vi "Measurement Logic2.vi"(8 "error in":errorcluster, 9 "measurement configuration":T2={"Capturing Stream"=FALSE, "Pause Capture In"=FALSE, "Interface Name In"="ENET9/monitor", "Update Interval s in"=0.2, "Packet Count"=0}, 10 "measure call context in":refnum<class "Measure Call Context.lvclass">) -> (0 "error out":errorcluster, 1 "measurement results":T1={"Dataframe"=[[""]], "Capturing Stream"=TRUE, "Packet Count Out"=0}, 2 "measure call context out":refnum<class "Measure Call Context.lvclass">)   [LabVIEW 2025, in "Automotive Ethernet Bus Monitor.lvclass"]
doc: "Contains the core logic for executing the measurement."
uses:
  Automotive Ethernet Bus Monitor.lvclass
  <vilib>/Plug-In SDKs/Measurements/Measure Call Context/Measure Call Context.lvclass
  Measurement Configuration.ctl
  Measurement Results.ctl
  <vilib>/xnet/xnet.llb/XNET Create Session (Frame Input Stream).vi
  <vilib>/xnet/xnet.llb/XNET Read (Frame Ethernet).vi
  <extravilib>/ChannelInstances/Event Messenger-bool/Instantiate.vi
  Automotive Ethernet Bus Monitor.lvclass/Automotive Ethernet Bus Monitor.ctl
  Program Files/NI/LVAddons/nixnet/1/examples/nixnet/projects/NI-XNET Ethernet/subVI/Ethernet.lvlib
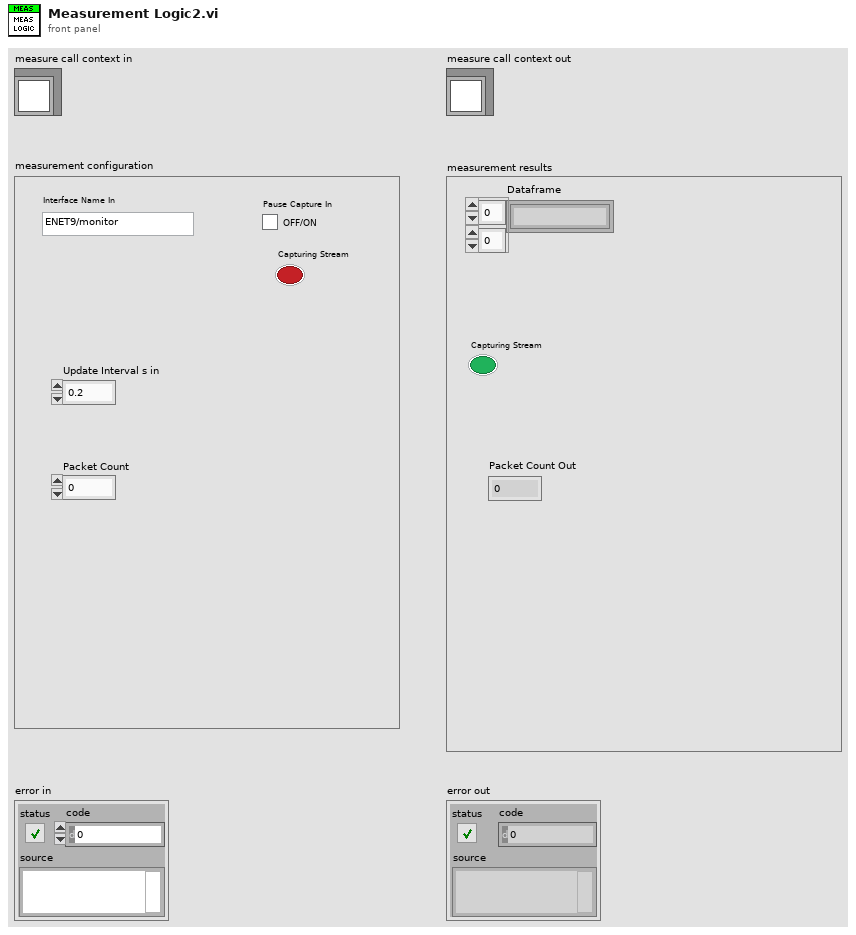
[diagram p1: front panel]
types:
  T1 = typedef "Automotive Ethernet Bus Monitor.lvclass/Measurement Results.ctl" = cluster{"Dataframe":string[][], "Capturing Stream":bool, "Packet Count Out":u32}
  T2 = typedef "Automotive Ethernet Bus Monitor.lvclass/Measurement Configuration.ctl" = cluster{"Capturing Stream":bool, "Pause Capture In":bool, "Interface Name In":string, "Update Interval s in":dbl, "Packet Count":u32}
  T3 = typedef "XNET Frame Ethernet.ctl" = cluster{"local timestamp":timestamp, "network timestamp":timestamp, "frame data":u8[], "fcs":u32, "type":T4, "network synced?":bool, "receive?":bool, "transmit?":bool, "error?":bool}
  T4 = typedef "XNET Frame Type Ethernet.ctl" = u16
  T5 = typedef "Ethernet.lvlib/Ethernet Header.ctl" = cluster{"destination MAC address":cluster{u8, u8, u8, u8, u8, u8}, "source MAC address":cluster{u8, u8, u8, u8, u8, u8}, "Has VLAN Tag":bool, "VLAN Tag":T6, "Ethertype":u16}
  T6 = typedef "Ethernet.lvlib/VLAN Tag.ctl" = cluster{"TPID":u16, "priority":u8, "DEI":bool, "VID":u16}
  T7 = typedef "Event Messenger-bool.lvlib/))Channel.ctl" = refnum<queue>
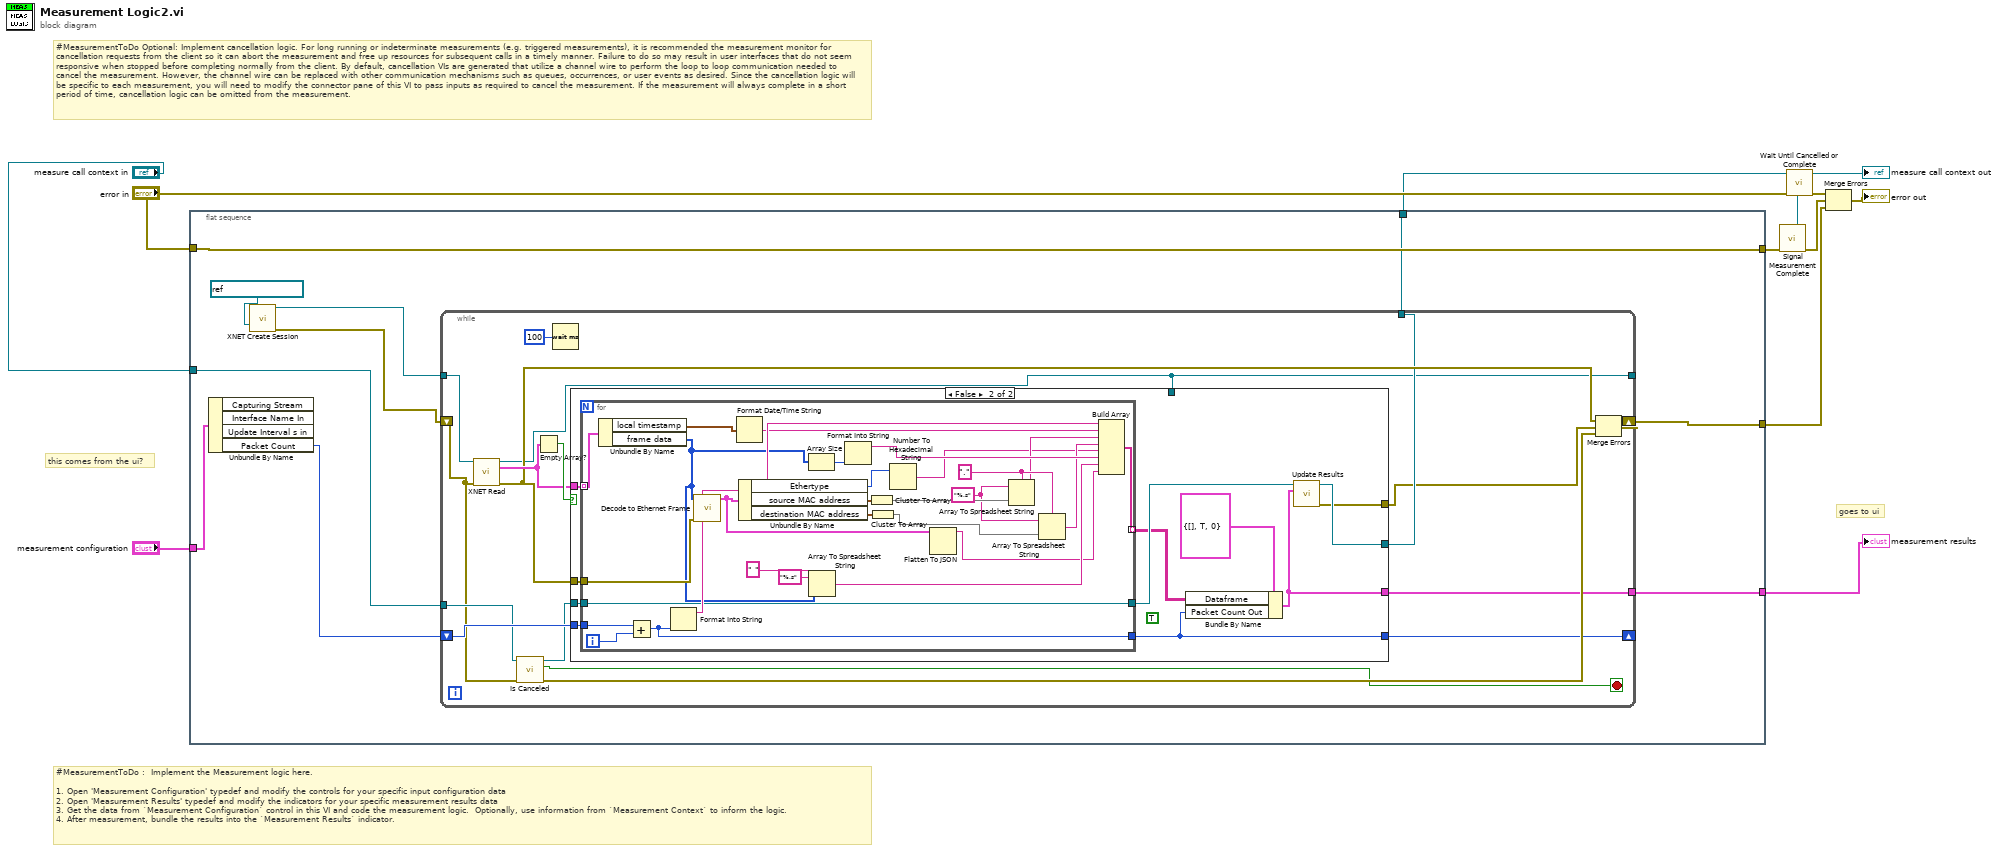
[diagram p0: block diagram]
diagram:
  # "goes to ui"
  # "this comes from the ui?"
  # "#MeasurementToDo Optional: Implement cancellation logic. For long running or indeterminate measurements (e.g. triggered measurements), it is recommended the measurement monitor for cancellation requests from the client so it can abort the measurement and free up resources for subsequent calls in a timely manner. Failure to do so may result in user interfaces that do not seem responsive when stopped before completing normally from the client. By default, cancellation VIs are generated that utilize a channel wire to perform the loop to loop communication needed to cancel the measurement. However, the channel wire can be replaced with other communication mechanisms such as queues, occurrences, or user events as desired. Since the cancellation logic will be specific to each measurement, you will need to modify the connector pane of this VI to pass inputs as required to cancel the measurement. If the measurement will always complete in a short period of time, cancellation logic can be omitted from the measurement."
  # "#MeasurementToDo :  Implement the Measurement logic here.\n\n1. Open 'Measurement Configuration' typedef and modify the controls for your specific input configuration data\n2. Open 'Measurement Results' typedef and modify the indicators for your specific measurement results data\n3. Get the data from `Measurement Configuration` control in this VI and code the measurement logic.  Optionally, use information from `Measurement Context` to inform the logic.\n4. After measurement, bundle the results into the `Measurement Results` indicator."
  n1 = flat-sequence {
    tunnel: "measurement configuration" -> [w21]
    tunnel: "error in" -> [w22]
    tunnel: [w22] -> w9
    tunnel: "measure call context in" -> [w18]
    tunnel: [w17] -> w3
    tunnel: [w16] -> w2
    tunnel: [w14] -> w1
    frame #0 {
      n2 = Unbundle By Name(w21) -> ("Packet Count"=w20:u32)  [unwired: 3 out]
      n3 = call-poly <vilib>:"XNET Create Session.vi"("interface"=refnum<k21> "ENET9/monitor") -> ("session out"=w15:refnum<k21>, "error out"=w13:errorcluster)  [unwired: 13 in]
      n4 = while {
        tunnel: w15 -> [w37]
        tunnel: [w25] -> _
        shift-right: [w26] -> _
        shift-left: w20 -> [w36]
        tunnel: w18 -> [w33]
        tunnel: [w30] -> w17
        tunnel: [w24] -> w14
        shift-right: [w34] -> w16
        shift-left: w13 -> [w23]
        stop <- w29 stop-if-true
        n5 = call-poly <vilib>:"XNET Read.vi"("session in"=w37, "error in (no error)"=w23) -> ("session out"=w25:refnum<k21>, "data"=w38:T3[], "error out"=w35:errorcluster)  [unwired: 10 in, 1 out]
        n6 = call <vilib>:"Is Canceled.vi"("error in"=w23, "measure call context in"=w33) -> ("error out"=w31:errorcluster, "is canceled?"=w29:bool, "measure call context out"=w32:refnum<class "Measure Call Context.lvclass">)  [unwired: 7 in]
        n7 = Empty Array?(array=w38) -> (empty?=w39:bool)
        n8 = Wait (ms)(milliseconds to wait=u32 100) -> ()  [unwired: 1 out]
        n9 = case shown="False" w39 {
          tunnel: w38 -> [_ w53]
          tunnel: w36 -> [w42 w52]
          tunnel: [w42 w45] -> w26
          tunnel: [w41 w49] -> w30
          tunnel: w35 -> [w40 w51]
          tunnel: w32 -> [w41 w50]
          tunnel: [w40 w48] -> w28
          tunnel: w25 -> [_ _]
          tunnel: [_ w44] -> w24
          frame True {
          }
          frame False {
            (unwired) TRUE ("Capturing Stream")
            n10 = for {
              tunnel: w53 -> [w81] mode=indexing
              tunnel: w52 -> [w72]
              tunnel: [w71] -> w45
              tunnel: w51 -> [w69]
              tunnel: w50 -> [w70]
              tunnel: [w70] -> w47
              tunnel: [w68] -> w43 mode=indexing
              i -> [w73]
              w64 = "%.s" ("format string")
              w65 = "." ("delimiter (Tab)")
              n11 = Unbundle By Name(w81) -> ("local timestamp"=w80:timestamp, "frame data"=w59:u8[])
              n12 = Add(x=w72, y=w73) -> (x+y=w71:u32)
              n13 = Format Into String(w71) -> (resulting string=w79:string)  [unwired: 3 in, 1 out]
              n14 = call "Decode to Ethernet Frame.vi"("error in (no error)"=w69, "frame data"=w59) -> ("Ethernet Header Cluster"=w54:T5)  [unwired: 7 in, 2 out]
              n15 = Format Date/Time String(seconds (now)=w80) -> (date/time string=w76:string)  [unwired: 2 in]
              n16 = Unbundle By Name(w54) -> ("Ethertype"=w56:u16, "source MAC address"=w78:cluster{u8, u8, u8, u8, u8, u8}, "destination MAC address"=w77:cluster{u8, u8, u8, u8, u8, u8})
              n17 = Array Size(array=w59) -> (size(s)=w75:i32)
              n18 = Array To Spreadsheet String(delimiter (Tab)=" ", array=w59, 3:"%.s" ("format string")) -> (spreadsheet string=w58:string)
              n19 = Format Into String(w75) -> (resulting string=w74:string)  [unwired: 3 in, 1 out]
              n20 = Cluster To Array(cluster=w78) -> (array=w67:u8[])
              n21 = Cluster To Array(cluster=w77) -> (array=w66:u8[])
              n22 = Number To Hexadecimal String(2:w56) -> (0:w57:string)  [unwired: 1 in]
              n23 = Flatten To JSON(anything=w54) -> (JSON string=w55:string)  [unwired: 2 in, 1 out]
              n24 = Array To Spreadsheet String(delimiter (Tab)=w65, array=w67, 3:w64) -> (spreadsheet string=w63:string)
              n25 = Array To Spreadsheet String(delimiter (Tab)=w65, array=w66, 3:w64) -> (spreadsheet string=w62:string)
              n26 = Build Array(w79, w76, w63, w62, w57, w74, w58, w55) -> (w68:string[])
            }
            n27 = Bundle By Name(cluster=T1 {"Dataframe"=[], "Capturing Stream"=TRUE, "Packet Count Out"=0} ("Measurement Results"), "Dataframe"=w43, "Packet Count Out"=w45) -> (w44:T1)
            n28 = call <vilib>:"Update Results.vi"("measurement results"=w44, "measure call context in"=w47) -> ("error out"=w48:errorcluster, "measure call context out"=w49:refnum<class "Measure Call Context.lvclass">)  [unwired: 8 in]
          }
        }
        n29 = Merge Errors(w35, w28, w31) -> (w34:errorcluster)
      }
    }
  }
  n30 = call "Signal Measurement Complete.vi"("error in (no error)"=w9) -> ("error out"=w7:errorcluster, "done channel"=w8:T7)  [unwired: 9 in]
  n31 = call "Wait Until Cancelled or Complete.vi"("done channel"=w8, "error in (no error)"="error in", "measure call context in"=w3) -> ("error out"=w6:errorcluster, "measure call context out"=→"measure call context out":refnum<class "Measure Call Context.lvclass">)  [unwired: 7 in]
  n32 = Merge Errors(w6, w7, w2) -> (→"error out":errorcluster)
  "measurement results" <- w1
